vi "Actuators Shutdown.vi"(11 "IO Cluster IN":T1) -> (3 "Error Out":errorcluster)   [LabVIEW 2019]
uses:
  Actuators IO Cluster.ctl
  <vilib>/Utility/error.llb/Error Cluster From Error Code.vi
  <vilib>/rvi/errors/niLvFpgaAdjustHostInterfaceError.vi
  <vilib>/FPGAPlugInAG/Dynamic/niLvFpga_Close_Dynamic.vi
  <vilib>/rvi/interface/nirviReadWriteControl/nirviReadWriteControl.xnode
  <vilib>/rvi/interface/nirviCloseFPGA/nirviCloseFPGA.xnode
  NiFpgaLv.dll
  <vilib>/rvi/interface/Simulation/niFpgaSimulationCallBeginRW.vi
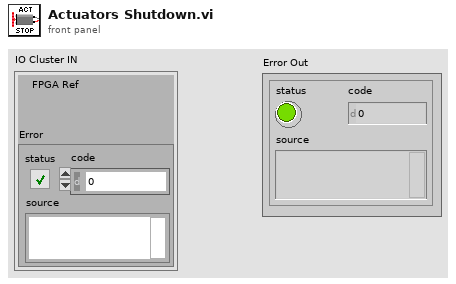
[diagram p1: front panel]
types:
  T1 = typedef "Actuators IO Cluster.ctl" = cluster{"Error":errorcluster, "FPGA Ref":refnum<k20>}
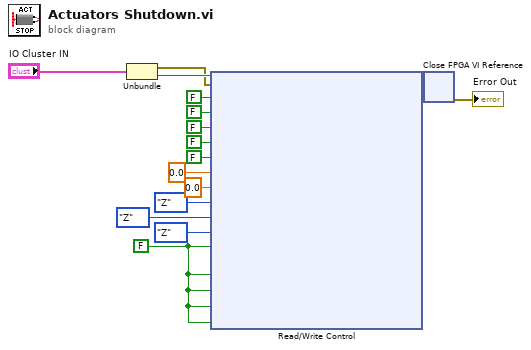
[diagram p0: block diagram]
diagram:
  w7 = FALSE ("LED DC Motor")
  n1 = Unbundle("IO Cluster IN") -> ("Error"=w2:errorcluster, "FPGA Ref"=w3:refnum<k20>)
  n2 = xnode "Read/Write Control"("FPGA VI引用输入"=w3, "错误输入"=w2, "Microstep Enable"=FALSE, "Stepper Control 1"=FALSE, "Stepper Control 2"=FALSE, "Stepper Control 3"=FALSE, "Stepper Control 4"=FALSE, "DC Linear Amplifier Value (+/-10)"=sgl 0.0, "DC Motor PWM (0-1)"=sgl 0.0, "BLDC Drive Phase A"=enum16{"H", "L", "Z"}."Z", "BLDC Drive Phase B"=enum16{"H", "L", "Z"}."Z", "BLDC Drive Phase C"=enum16{"H", "L", "Z"}."Z", "LED DC Motor"=w7, "LED BLDC"=w7, "LED Stepper"=w7, "LED Servo"=w7, "LED Status"=w7) -> ("FPGA VI引用输出"=w5:refnum<k20>, "错误输出"=w6:errorcluster)
  n3 = xnode "Close FPGA VI Reference"("FPGA VI Reference In"=w5, "error in"=w6) -> ("error out"=→"Error Out":errorcluster)
